vi "LogLoop.vi"(8 "Error In":errorcluster, 9 "Executable Configuration":T1, 10 "Data Structures":T2, 11 "Action Queues":T3) -> (0 "Error Out":errorcluster)   [LabVIEW 2012]
uses:
  ActionQueues.ctl
  UIActionQueueElement.ctl
  UIAction.ctl
  HardwareActionQueueElement.ctl
  HardwareAction.ctl
  LogActionQueueElement.ctl
  LogAction.ctl
  DataStructures.ctl
  HardwareDisplayData.ctl
  HardwareLogData.ctl
  ExecutableConfiguration.ctl
  Setup.ctl
  DUTConfiguration.ctl
  driver/Public/Controls/SMUSense.ctl
  LogConfiguration.ctl
  LogStartConfiguration.ctl
  LogStartTriggerType.ctl
  LogDigitalIOTriggerEdge.ctl
  LogRolloverConfiguration.ctl
  LogRolloverTriggerType.ctl
  LogStopConfiguration.ctl
  LogStopTriggerType.ctl
  TriggerConfiguration.ctl
  TriggerInputConfiguration.ctl
  TriggerInputType.ctl
  driver/Public/Controls/TriggerMode.ctl
  TriggerOutputConfiguration.ctl
  TriggerOutputType.ctl
  SourceConfiguration.ctl
  SourceFunction.ctl
  MeasureConfiguration.ctl
  LogStartTimeGlobalAction.ctl
  LogFileGlobalAction.ctl
  driver/Keithley-2602.lvlib
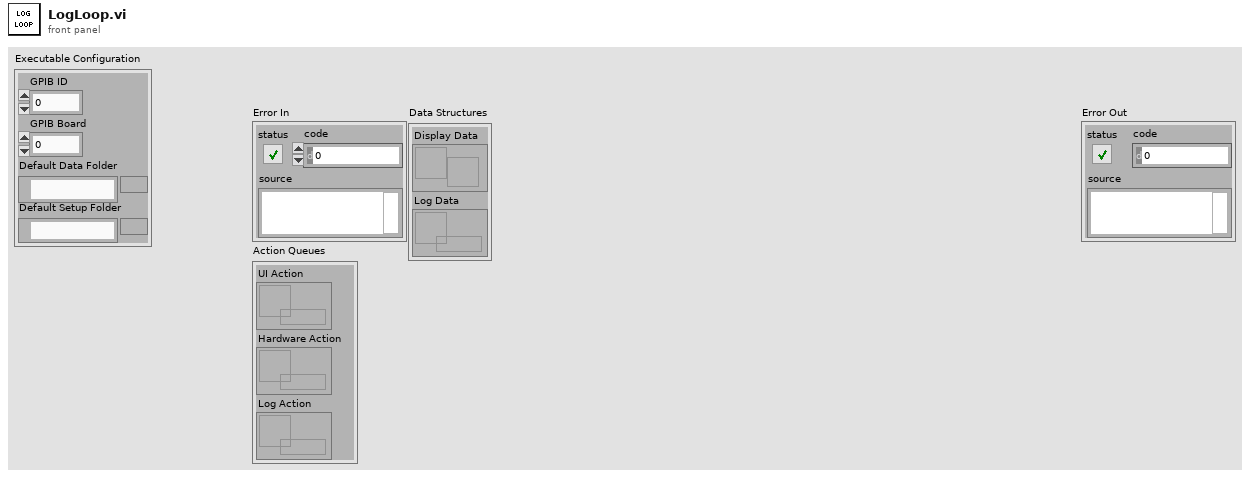
[diagram p1: front panel]
types:
  T1 = typedef "ExecutableConfiguration.ctl" = cluster{"GPIB ID":u8, "GPIB Board":u8, "Default Data Folder":path, "Default Setup Folder":path}
  T2 = typedef "DataStructures.ctl" = cluster{"Display Data":refnum<notifier>, "Log Data":refnum<queue>}
  T3 = typedef "ActionQueues.ctl" = cluster{"UI Action":refnum<queue>, "Hardware Action":refnum<queue>, "Log Action":refnum<queue>}
  T4 = typedef "Setup.ctl" = cluster{"DUT":T5, "Log":T7, "Trigger":T15, "Sources":T21[], "Measures":T23[]}
  T5 = typedef "DUTConfiguration.ctl" = cluster{"Count":u32, "Wirings":T6[], "Names":string[][]}
  T6 = typedef "Keithley-2602.lvlib/SMUSense.ctl" = enum16{"Local (2-wire)", "Remote (4-wire)", "Calibration"}
  T7 = typedef "LogConfiguration.ctl" = cluster{"Start":T8, "Rollover":T11, "Stop":T13}
  T8 = typedef "LogStartConfiguration.ctl" = cluster{"Trigger Type":T9, "Timer (sec)":dbl, "Digital IO Line":u8, "Digital IO Edge":T10}
  T9 = typedef "LogStartTriggerType.ctl" = enum16{"Immediate", "User", "Timer", "Digital IO"}
  T10 = typedef "LogDigitalIOTriggerEdge.ctl" = enum16{"Rising", "Falling"}
  T11 = typedef "LogRolloverConfiguration.ctl" = cluster{"Trigger Type":T12, "Timer (sec)":dbl, "File Size (MB)":u32, "Digital IO Line":u8, "Digital IO Edge":T10}
  T12 = typedef "LogRolloverTriggerType.ctl" = enum16{"None", "Timer", "File Size", "Digital IO"}
  T13 = typedef "LogStopConfiguration.ctl" = cluster{"Trigger Type":T14, "Timer (sec)":dbl, "File Size (MB)":u32, "Digital IO Line":u8, "Digital IO Edge":T10}
  T14 = typedef "LogStopTriggerType.ctl" = enum16{"None", "User", "Timer", "File Size", "Digital IO"}
  T15 = typedef "TriggerConfiguration.ctl" = cluster{"Input":T16, "Output":T19}
  T16 = typedef "TriggerInputConfiguration.ctl" = cluster{"Type":T17, "Timeout (ms)":u32, "Delay (ms)":u32, "Digital IO Line (1-14)":u8, "Digital IO Mode":T18}
  T17 = typedef "TriggerInputType.ctl" = enum16{"None", "Digital IO", "Bus"}
  T18 = typedef "Keithley-2602.lvlib/TriggerMode.ctl" = enum16{"Falling", "Rising", "Either", "Synchronous"}
  T19 = typedef "TriggerOutputConfiguration.ctl" = cluster{"Type":T20, "Delay (ms)":u32, "Digital IO Line (1-14)":u8, "Digital IO Mode":T18, "Digital IO Pulse Width (sec)":dbl}
  T20 = typedef "TriggerOutputType.ctl" = enum16{"None", "Digital IO", "Bus"}
  T21 = typedef "SourceConfiguration.ctl" = cluster{"Enabled?":bool, "Function":T22, "Level (V or A)":dbl, "Autorange Enabled?":bool, "High Limit (V or A)":dbl, "Low Limit (V or A)":dbl}
  T22 = typedef "SourceFunction.ctl" = enum16{"Voltage", "Current"}
  T23 = typedef "MeasureConfiguration.ctl" = cluster{"Enabled?":bool, "Count":u8, "Interval (sec)":dbl, "Voltage Auto Range Enabled?":bool, "Voltage High Limit (V or A)":dbl, "Voltage Low Limit (V or A)":dbl, "Current Auto Range Enabled?":bool, "Current High Limit (V or A)":dbl, "Current Low Limit (V or A)":dbl}
  T24 = typedef "LogStartTimeGlobalAction.ctl" = enum16{"Set", "Get"}
  T25 = typedef "LogActionQueueElement.ctl" = cluster{"Action":T26, "Data":variant}
  T26 = typedef "LogAction.ctl" = enum16{"Initialize", "Start", "Arm", "Create", "Write", "Close", "Rearm", "Stop", "Error", "Shutdown"}
  T27 = typedef "UIActionQueueElement.ctl" = cluster{"Action":T28, "Data":variant}
  T28 = typedef "UIAction.ctl" = enum16{"Initialize", "Configure Trigger", "Configure Measure", "Configure Source", "Configure DUT", "Configure Log", "Configure Open", "Configure Save", "Configure Reset", "Hardware Start", "Hardware Started", "Hardware Stop", "Hardware Stopped", "Log Arm", "Log Start", "Log Started", "Log Stop", "Log Stopped", "Error", "Shutdown"}
  T29 = typedef "LogFileGlobalAction.ctl" = enum16{"Open", "Write", "Size", "Close"}
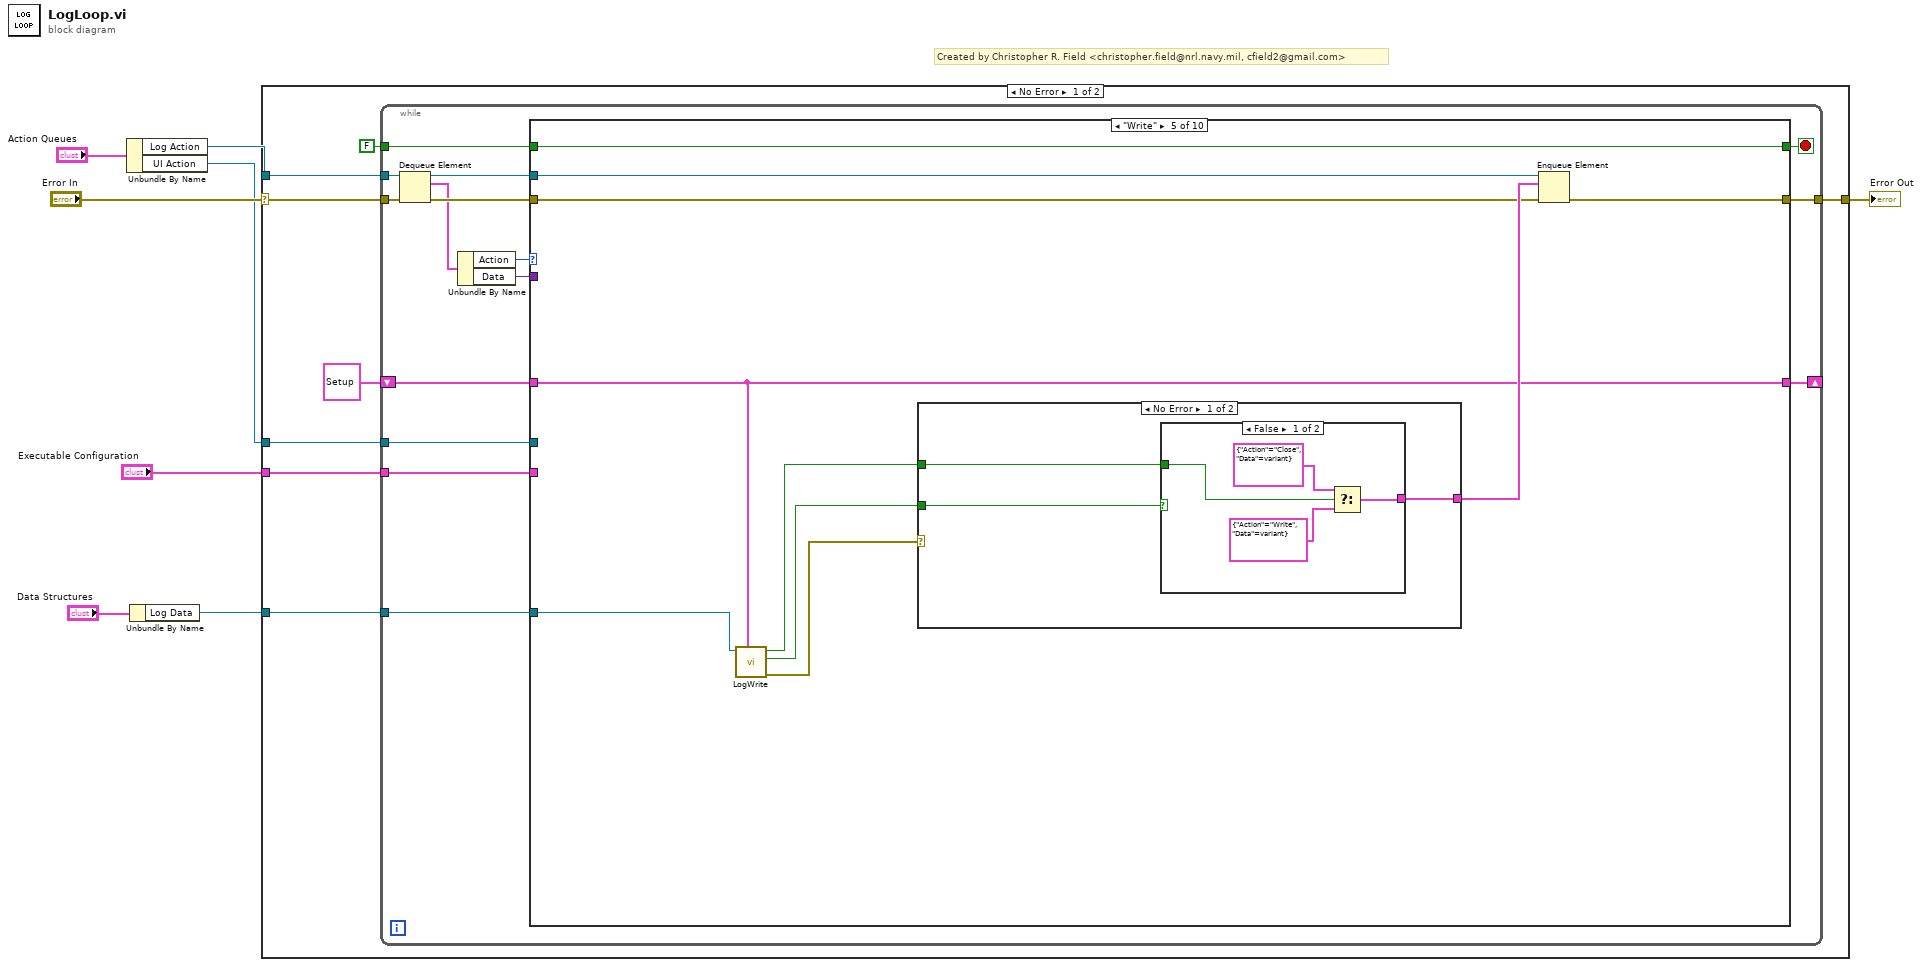
[diagram p0: block diagram]
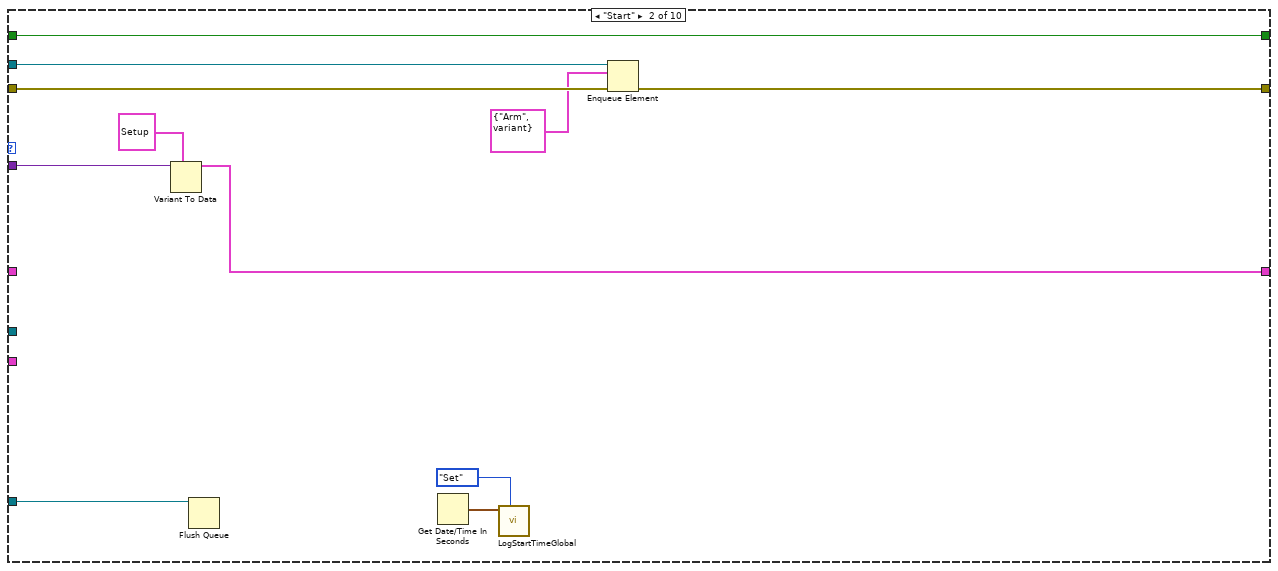
[diagram p3: hidden frame]
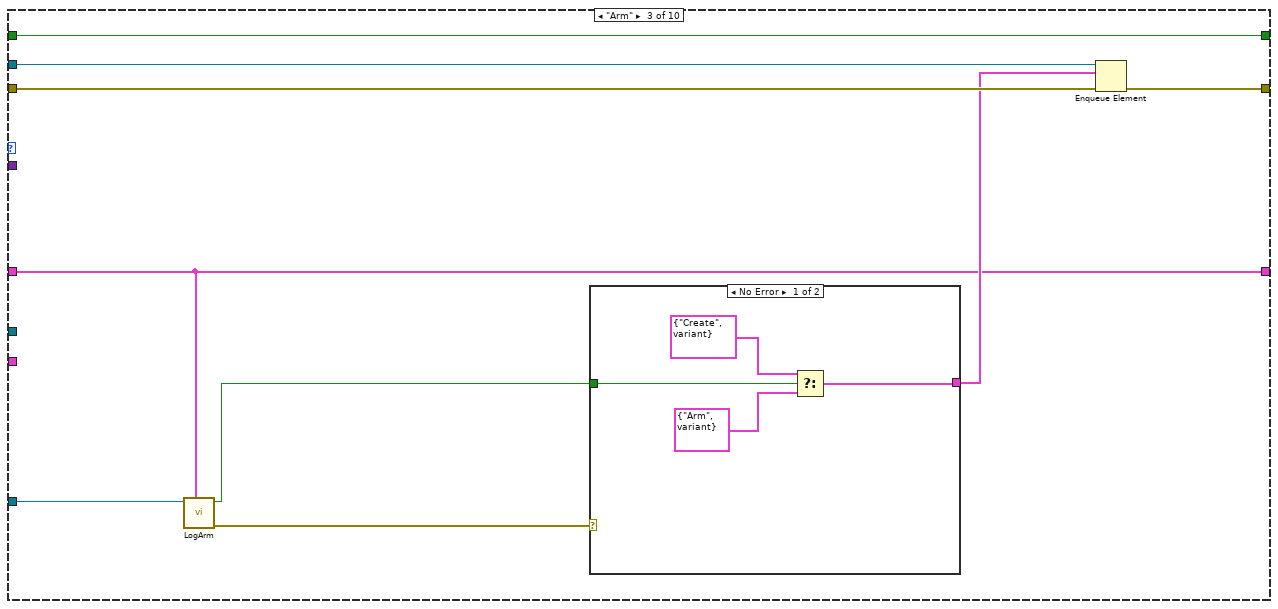
[diagram p4: hidden frame]
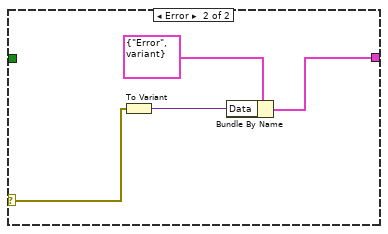
[diagram p5: hidden frame]
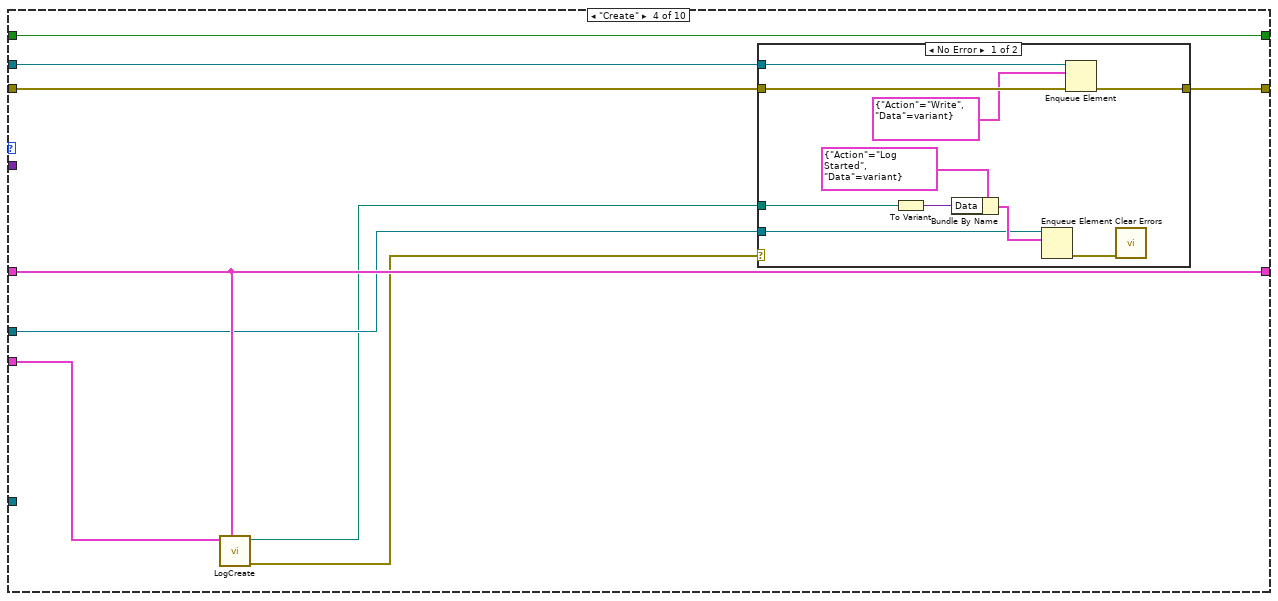
[diagram p6: hidden frame]
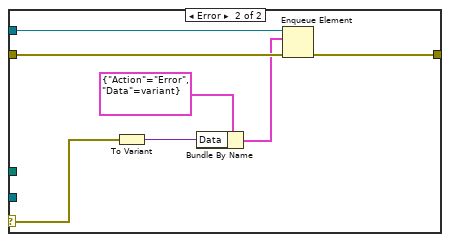
[diagram p7: hidden frame]
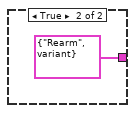
[diagram p8: hidden frame]
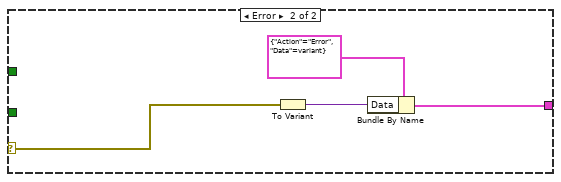
[diagram p9: hidden frame]
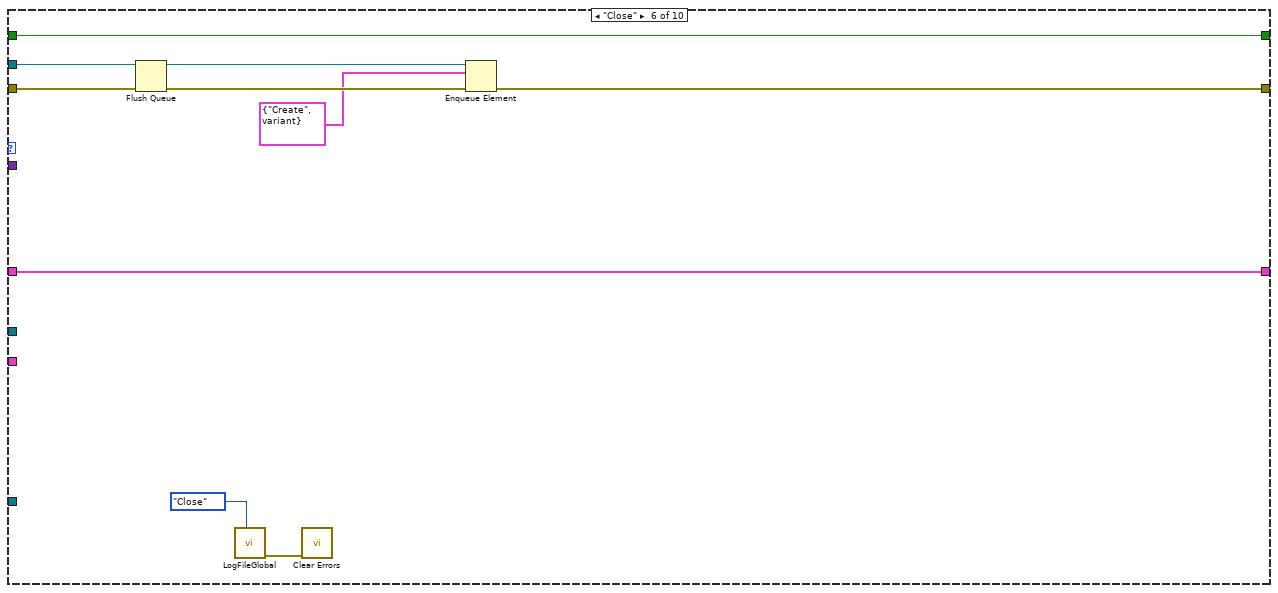
[diagram p10: hidden frame]
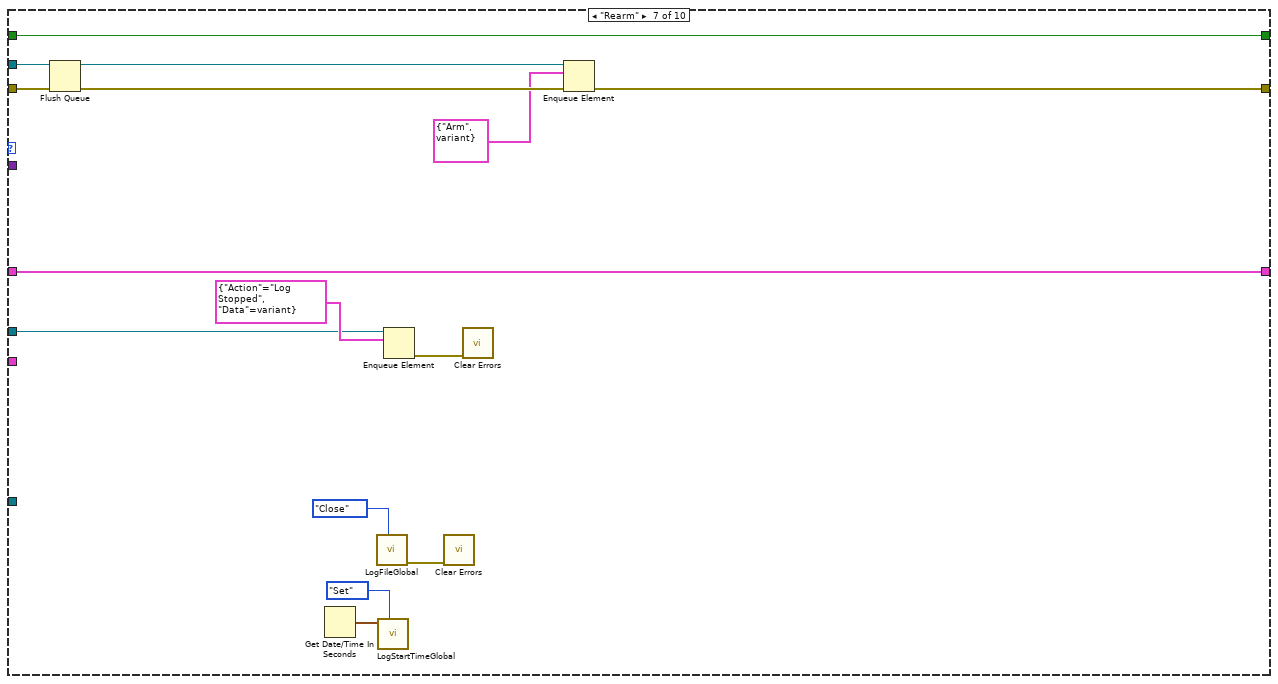
[diagram p11: hidden frame]
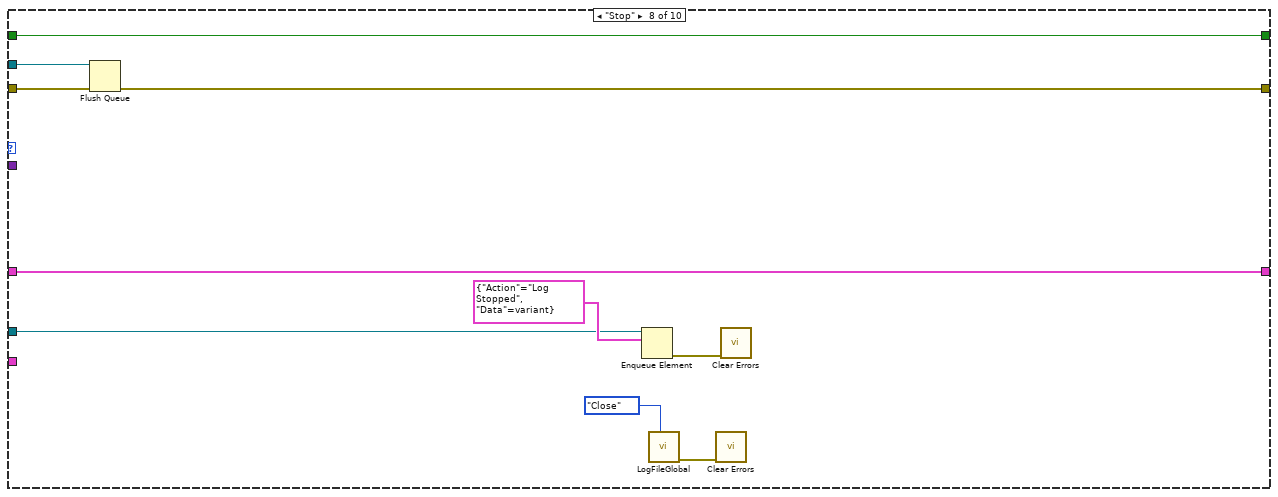
[diagram p12: hidden frame]
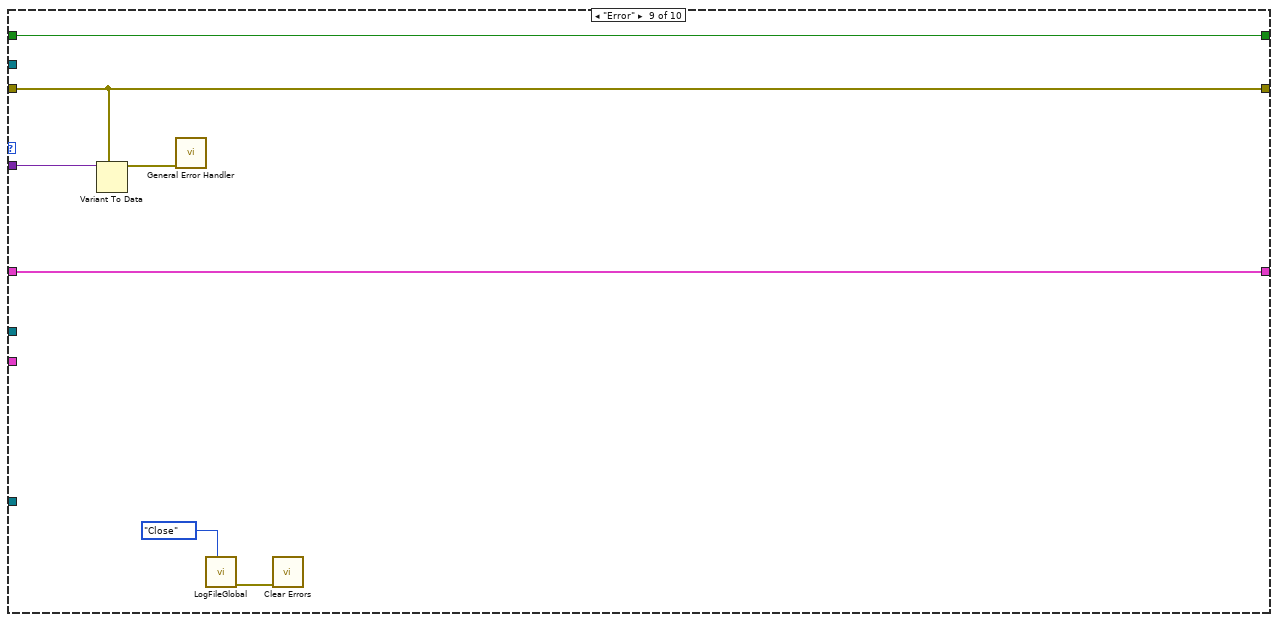
[diagram p13: hidden frame]
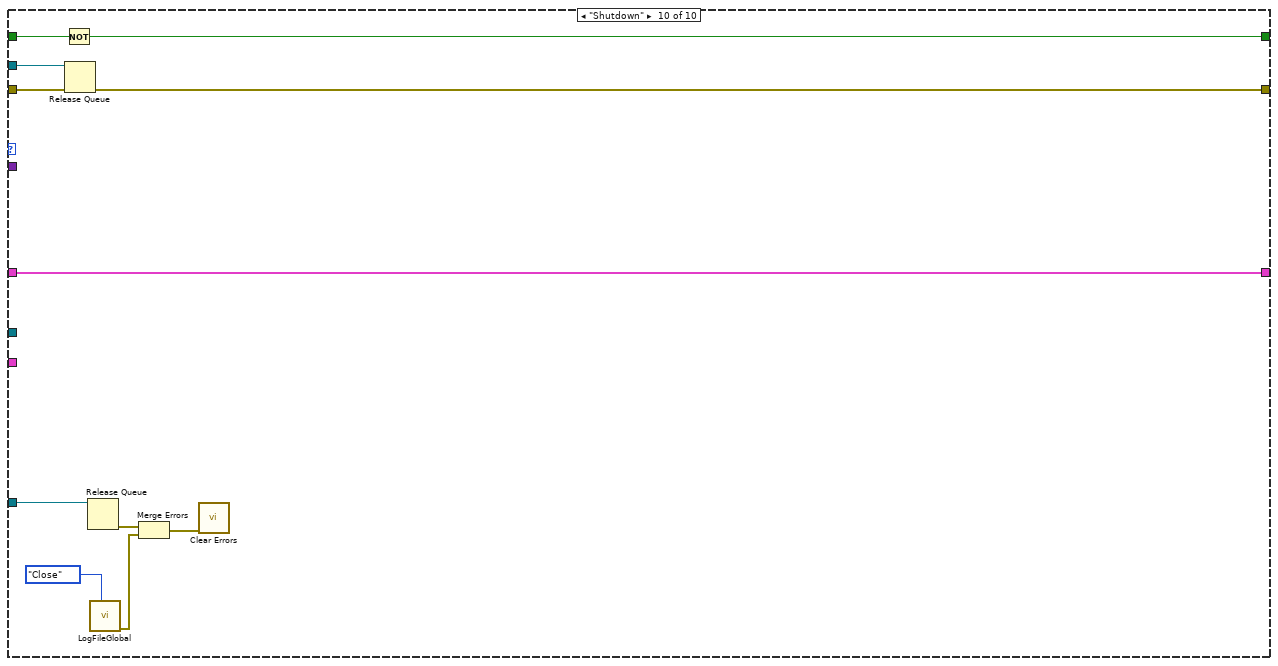
[diagram p14: hidden frame]
diagram:
  # "Created by Christopher R. Field <christopher.field@nrl.navy.mil, cfield2@gmail.com>"
  n1 = Unbundle By Name("Action Queues") -> ("Log Action"=w4:refnum<queue>, "UI Action"=w3:refnum<queue>)
  n2 = Unbundle By Name("Data Structures") -> ("Log Data"=w1:refnum<queue>)
  n3 = case shown="No Error" "Error In" {
    selector: "Error In" -> [w16 w164]
    tunnel: [w13 w164] -> w7
    tunnel: w4 -> [w14 _]
    tunnel: "Executable Configuration" -> [w12 _]
    tunnel: w3 -> [w11 _]
    tunnel: w1 -> [w10 _]
    frame No Error {
      n4 = while {
        tunnel: w16 -> [w31]
        tunnel: FALSE -> [w30]
        tunnel: w14 -> [w28]
        tunnel: [w22] -> w13
        tunnel: w12 -> [w21]
        tunnel: w11 -> [w20]
        tunnel: w10 -> [w19]
        shift-right: [w18] -> _
        shift-left: T4 {"DUT"={"Count"=1, "Wirings"=[], "Names"=[]}, "Log"={"Start"={"Trigger Type"=enum."Immediate", "Timer (sec)"=0.0, "Digital IO Line"=0, "Digital IO Edge"=enum."Rising"}, "Rollover"={"Trigger Type"=enum."None", "Timer (sec)"=0.0, "File Size (MB)"=0, "Digital IO Line"=0, "Digital IO Edge"=enum."Rising"}, "Stop"={"Trigger Type"=enum."None", "Timer (sec)"=0.0, "File Size (MB)"=0, "Digital IO Line"=0, "Digital IO Edge"=enum."Rising"}}, "Trigger"={"Input"={"Type"=enum."None", "Timeout (ms)"=0, "Delay (ms)"=0, "Digital IO Line (1-14)"=0, "Digital IO Mode"=enum."Falling"}, "Output"={"Type"=enum."None", "Delay (ms)"=0, "Digital IO Line (1-14)"=0, "Digital IO Mode"=enum."Falling", "Digital IO Pulse Width (sec)"=0.0}}, "Sources"=[], "Measures"=[]} ("Application Configuration") -> [w17]
        stop <- w23 stop-if-true
        n5 = Dequeue Element(queue=w28, error in (no error)=w31) -> (queue out=w27:refnum<queue>, element=w26:T25, error out=w29:errorcluster)  [unwired: 1 in, 1 out]
        n6 = Unbundle By Name(w26) -> ("Action"=w25:T26, "Data"=w24:variant)
        n7 = case shown="\"Write\"" w25 {
          tunnel: w30 -> [w33 w40 w54 w71 w98 w120 w131 w142 w152 w160]
          tunnel: w29 -> [w34 w42 w52 w70 w92 w118 w132 w144 w149 w162]
          tunnel: w27 -> [_ w43 w53 w68 w93 w119 w133 w145 _ w163]
          tunnel: w24 -> [_ w44 _ _ _ _ _ _ w150 _]
          tunnel: [w33 w40 w54 w71 w98 w120 w131 w142 w152 w159] -> w23
          tunnel: [w34 w41 w51 w69 w97 w115 w127 w143 w149 w161] -> w22
          tunnel: w21 -> [_ _ _ w67 _ _ _ _ _ _]
          tunnel: w20 -> [_ _ _ w64 _ _ w134 w136 _ _]
          tunnel: w19 -> [_ w37 w49 _ w91 _ _ _ _ w158]
          tunnel: [w32 w38 w48 w66 w95 w114 w130 w141 w151 w157] -> w18
          tunnel: w17 -> [w32 _ w48 w66 w95 w114 w130 w141 w151 w157]
          frame "Initialize", Default {
          }
          frame "Start" {
            n8 = Variant To Data(type=T4 {"DUT"={"Count"=1, "Wirings"=[], "Names"=[]}, "Log"={"Start"={"Trigger Type"=enum."Immediate", "Timer (sec)"=0.0, "Digital IO Line"=0, "Digital IO Edge"=enum."Rising"}, "Rollover"={"Trigger Type"=enum."None", "Timer (sec)"=0.0, "File Size (MB)"=0, "Digital IO Line"=0, "Digital IO Edge"=enum."Rising"}, "Stop"={"Trigger Type"=enum."None", "Timer (sec)"=0.0, "File Size (MB)"=0, "Digital IO Line"=0, "Digital IO Edge"=enum."Rising"}}, "Trigger"={"Input"={"Type"=enum."None", "Timeout (ms)"=0, "Delay (ms)"=0, "Digital IO Line (1-14)"=0, "Digital IO Mode"=enum."Falling"}, "Output"={"Type"=enum."None", "Delay (ms)"=0, "Digital IO Line (1-14)"=0, "Digital IO Mode"=enum."Falling", "Digital IO Pulse Width (sec)"=0.0}}, "Sources"=[], "Measures"=[]} ("Application Configuration"), Variant=w44) -> (data=w38:T4)  [unwired: 1 in, 1 out]
            n9 = Flush Queue(queue=w37) -> ()  [unwired: 1 in, 3 out]
            n10 = Get Date/Time In Seconds() -> (seconds since 1Jan1904=w35:timestamp)
            n11 = call "LogStartTimeGlobal.vi"("Action"=LogStartTimeGlobalAction."Set", "Set Value"=w35) -> ()  [unwired: 9 in, 1 out]
            n12 = Enqueue Element(queue=w43, element=T25 {"Action"=enum."Arm", "Data"=variant}, error in (no error)=w42) -> (error out=w41:errorcluster)  [unwired: 1 in, 2 out]
          }
          frame "Arm" {
            n13 = call "LogArm.vi"("Application Configuration"=w48, "Log Data In"=w49) -> ("Error Out"=w46:errorcluster, "Triggered?"=w47:bool)  [unwired: 8 in]
            n14 = case shown="No Error" w46 {
              selector: w46 -> [_ w60]
              tunnel: [w56 w59] -> w50
              tunnel: w47 -> [w55 _]
              frame No Error {
                n15 = Select(t=T25 {"Action"=enum."Create", "Data"=variant} ("element"), s=w55, f=T25 {"Action"=enum."Arm", "Data"=variant} ("element")) -> (s? t:f=w56:T25)
              }
              frame Error {
                n16 = To Variant(anything=w60) -> (Variant=w61:variant)
                n17 = Bundle By Name(cluster=T25 {"Action"=enum."Error", "Data"=variant} ("element"), "Data"=w61) -> (w59:T25)
              }
            }
            n18 = Enqueue Element(queue=w53, element=w50, error in (no error)=w52) -> (error out=w51:errorcluster)  [unwired: 1 in, 2 out]
          }
          frame "Create" {
            n19 = call "LogCreate.vi"("Application Configuration"=w66, "Executable Configuration"=w67) -> ("Error Out"=w65:errorcluster, "Log File"=w63:path)  [unwired: 8 in]
            n20 = case shown="No Error" w65 {
              selector: w65 -> [_ w83]
              tunnel: w70 -> [w81 w87]
              tunnel: [w80 w86] -> w69
              tunnel: w68 -> [w79 w88]
              tunnel: w64 -> [w74 _]
              tunnel: w63 -> [w72 _]
              frame No Error {
                n21 = To Variant(anything=w72) -> (Variant=w76:variant)
                n22 = Bundle By Name(cluster=T27 {"Action"=enum."Log Started", "Data"=variant} ("element"), "Data"=w76) -> (w75:T27)
                n23 = Enqueue Element(queue=w74, element=w75) -> (error out=w73:errorcluster)  [unwired: 2 in, 2 out]
                n24 = Enqueue Element(queue=w79, element=T25 {"Action"=enum."Write", "Data"=variant}, error in (no error)=w81) -> (error out=w80:errorcluster)  [unwired: 1 in, 2 out]
                n25 = call <vilib>:"Clear Errors.vi"("error in (no error)"=w73) -> ()  [unwired: 6 in, 1 out]
              }
              frame Error {
                n26 = To Variant(anything=w83) -> (Variant=w84:variant)
                n27 = Bundle By Name(cluster=T25 {"Action"=enum."Error", "Data"=variant} ("element"), "Data"=w84) -> (w82:T25)
                n28 = Enqueue Element(queue=w88, element=w82, error in (no error)=w87) -> (error out=w86:errorcluster)  [unwired: 1 in, 2 out]
              }
            }
          }
          frame "Write" {
            n29 = call "LogWrite.vi"("Application Configuration"=w95, "Log Data"=w91) -> ("Error Out"=w94:errorcluster, "Rearm?"=w89:bool, "Rollover?"=w90:bool)  [unwired: 7 in]
            n30 = case shown="No Error" w94 {
              selector: w94 -> [_ w107]
              tunnel: [w101 w108] -> w96
              tunnel: w90 -> [w100 _]
              tunnel: w89 -> [w99 _]
              frame No Error {
                n31 = case shown="False" w99 {
                  tunnel: [w103 T25 {"Action"=enum."Rearm", "Data"=variant} ("element")] -> w101
                  tunnel: w100 -> [w102 _]
                  frame False {
                    n32 = Select(t=T25 {"Action"=enum."Close", "Data"=variant} ("element"), s=w102, f=T25 {"Action"=enum."Write", "Data"=variant} ("element")) -> (s? t:f=w103:T25)
                  }
                  frame True {
                  }
                }
              }
              frame Error {
                n33 = To Variant(anything=w107) -> (Variant=w109:variant)
                n34 = Bundle By Name(cluster=T25 {"Action"=enum."Error", "Data"=variant} ("element"), "Data"=w109) -> (w108:T25)
              }
            }
            n35 = Enqueue Element(queue=w93, element=w96, error in (no error)=w92) -> (error out=w97:errorcluster)  [unwired: 1 in, 2 out]
          }
          frame "Close" {
            n36 = Flush Queue(queue=w119, error in (no error)=w118) -> (queue out=w117:refnum<queue>, error out=w116:errorcluster)  [unwired: 1 out]
            n37 = call "LogFileGlobal.vi"("Action"=LogFileGlobalAction."Close") -> ("Error Out"=w111:errorcluster)  [unwired: 9 in, 1 out]
            n38 = call <vilib>:"Clear Errors.vi"("error in (no error)"=w111) -> ()  [unwired: 6 in, 1 out]
            n39 = Enqueue Element(queue=w117, element=T25 {"Action"=enum."Create", "Data"=variant}, error in (no error)=w116) -> (error out=w115:errorcluster)  [unwired: 1 in, 2 out]
          }
          frame "Rearm" {
            n40 = Flush Queue(queue=w133, error in (no error)=w132) -> (queue out=w129:refnum<queue>, error out=w128:errorcluster)  [unwired: 1 out]
            n41 = Get Date/Time In Seconds() -> (seconds since 1Jan1904=w121:timestamp)
            n42 = call "LogFileGlobal.vi"("Action"=LogFileGlobalAction."Close") -> ("Error Out"=w123:errorcluster)  [unwired: 9 in, 1 out]
            n43 = call "LogStartTimeGlobal.vi"("Action"=LogStartTimeGlobalAction."Set", "Set Value"=w121) -> ()  [unwired: 9 in, 1 out]
            n44 = Enqueue Element(queue=w134, element=T27 {"Action"=enum."Log Stopped", "Data"=variant}) -> (error out=w125:errorcluster)  [unwired: 2 in, 2 out]
            n45 = call <vilib>:"Clear Errors.vi"("error in (no error)"=w123) -> ()  [unwired: 6 in, 1 out]
            n46 = call <vilib>:"Clear Errors.vi"("error in (no error)"=w125) -> ()  [unwired: 6 in, 1 out]
            n47 = Enqueue Element(queue=w129, element=T25 {"Action"=enum."Arm", "Data"=variant}, error in (no error)=w128) -> (error out=w127:errorcluster)  [unwired: 1 in, 2 out]
          }
          frame "Stop" {
            n48 = Flush Queue(queue=w145, error in (no error)=w144) -> (error out=w143:errorcluster)  [unwired: 2 out]
            n49 = Enqueue Element(queue=w136, element=T27 {"Action"=enum."Log Stopped", "Data"=variant}) -> (error out=w139:errorcluster)  [unwired: 2 in, 2 out]
            n50 = call "LogFileGlobal.vi"("Action"=LogFileGlobalAction."Close") -> ("Error Out"=w137:errorcluster)  [unwired: 9 in, 1 out]
            n51 = call <vilib>:"Clear Errors.vi"("error in (no error)"=w137) -> ()  [unwired: 6 in, 1 out]
            n52 = call <vilib>:"Clear Errors.vi"("error in (no error)"=w139) -> ()  [unwired: 6 in, 1 out]
          }
          frame "Error" {
            n53 = Variant To Data(type=w149, Variant=w150) -> (data=w148:errorcluster)  [unwired: 1 in, 1 out]
            n54 = call <vilib>:"General Error Handler.vi"("error in (no error)"=w148) -> ()  [unwired: 10 in, 5 out]
            n55 = call "LogFileGlobal.vi"("Action"=LogFileGlobalAction."Close") -> ("Error Out"=w146:errorcluster)  [unwired: 9 in, 1 out]
            n56 = call <vilib>:"Clear Errors.vi"("error in (no error)"=w146) -> ()  [unwired: 6 in, 1 out]
          }
          frame "Shutdown" {
            n57 = Not(x=w160) -> (.not. x?=w159:bool)
            n58 = Release Queue(queue=w163, error in (no error)=w162) -> (error out=w161:errorcluster)  [unwired: 1 in, 2 out]
            n59 = Release Queue(queue=w158) -> (error out=w156:errorcluster)  [unwired: 2 in, 2 out]
            n60 = call "LogFileGlobal.vi"("Action"=LogFileGlobalAction."Close") -> ("Error Out"=w153:errorcluster)  [unwired: 9 in, 1 out]
            n61 = Merge Errors(w156, w153) -> (w155:errorcluster)
            n62 = call <vilib>:"Clear Errors.vi"("error in (no error)"=w155) -> ()  [unwired: 6 in, 1 out]
          }
        }
      }
    }
    frame Error {
    }
  }
  "Error Out" <- w7
